vi "ArrayFile.vi"(11 "File Path":string) -> (0 "error out":errorcluster, 3 "Array":dbl[](array[numeric]))   [LabVIEW 2023]
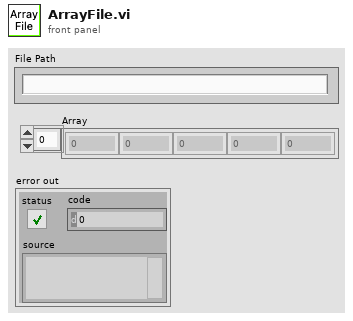
[diagram p1: front panel]
types:
  T1 = enum16{"open", "replace", "create", "open or create", "replace or create", "replace or create with confirmation"}
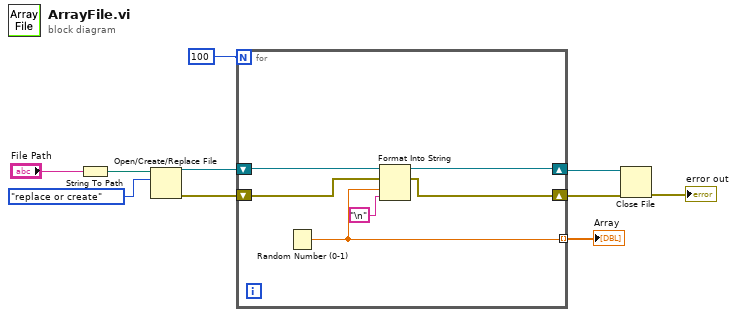
[diagram p0: block diagram]
diagram:
  n1 = String To Path(string="File Path") -> (path=w5:path)
  n2 = Open/Create/Replace File(file path (use dialog)=w5, operation (0:open)=T1."replace or create") -> (refnum out=w9:refnum<file>, error out=w10:errorcluster)  [unwired: 4 in, 1 out]
  n3 = for {
    N: 100 -> [_]
    shift-right: [w14] -> w2
    shift-left: w10 -> [w13]
    shift-right: [w15] -> w3
    shift-left: w9 -> [w16]
    tunnel: [w11] -> w8 mode=indexing
    n4 = Random Number (0-1)() -> (number: 0 to 1=w11:dbl)
    n5 = Format Into String(initial string=w16, error in=w13, w11, "\n") -> (resulting string=w15:refnum<file>, error out=w14:errorcluster)  [unwired: 1 in]
  }
  "Array" <- w8
  n6 = Close File(refnum=w3, error in=w2) -> (error out=→"error out":errorcluster)  [unwired: 1 out]
